vi "Robot Global Data.vi"() -> ()   [LabVIEW 2013]
doc: "This global VI can contain as many global variables as you need. Place a control on the panel, give it a good name. To read or write to it from a VI, drag the icon to the diagram of that VI. You can also drag from the project. Click on the node to change which global you access. You shouldn't have multiple locations writing to a global or it will cause a race-condition."
uses:
  <vilib>/Rock Robotics/WPI/Camera/WPI_CameraImageSize.ctl
panel:
  out "Target Info":T1(array[cluster])
  in  "LED toggle rate (ms)":u32=20
  in  "image size":T2=enum."320x240"
  in  "Enable Vision":bool
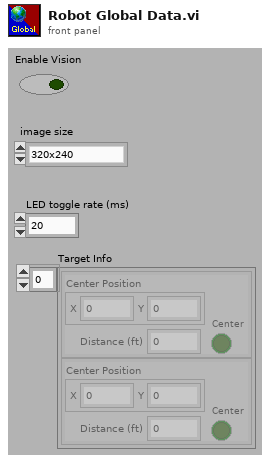
[diagram p1: front panel]
types:
  T1 = cluster{"Center Position":cluster{"X":dbl, "Y":dbl}, "Distance (ft)":dbl, "Center":bool}[]
  T2 = typedef "WPI_CameraImageSize.ctl" = enum16{"640x480", "320x240", "160x120"}
diagram:
